vi "例6-18.vi"() -> ()   [LabVIEW 2019]
uses:
  <vilib>/Analysis/4window.llb/Hanning Window (DBL).vi
  <vilib>/Analysis/4window.llb/AllCosWindow (DBL).vi
  <vilib>/Analysis/NI_AALBase.lvlib
  <vilib>/Analysis/NI_AALPro.lvlib
panel:
  in  "停止":bool
  in  "信号2幅值":dbl=1.0
  in  "信号2频率":dbl=48.67
  in  "信号1幅值":dbl=0.001
  in  "信号1频率":dbl=90.2
  out "频谱图":dbl[][](graph)
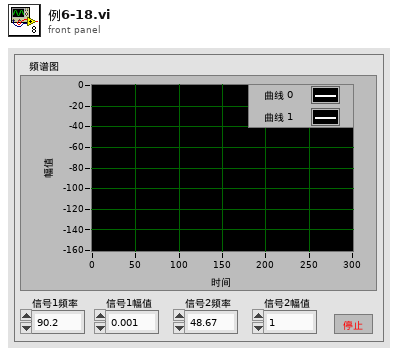
[diagram p1: front panel]
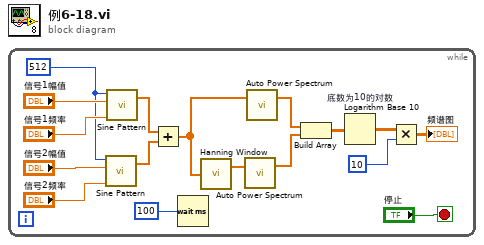
[diagram p0: block diagram]
diagram:
  n1 = while {
    stop <- "停止" stop-if-true
    w15 = 512
    n2 = call <vilib>:"Sine Pattern.vi"("cycles"="信号2频率", "amplitude"="信号2幅值", "samples"=w15) -> ("Sinusoidal Pattern"=w11:dbl[])  [unwired: 1 in, 1 out]
    n3 = call <vilib>:"Sine Pattern.vi"("cycles"="信号1频率", "amplitude"="信号1幅值", "samples"=w15) -> ("Sinusoidal Pattern"=w12:dbl[])  [unwired: 1 in, 1 out]
    n4 = Add(x=w12, y=w11) -> (x+y=w10:dbl[])
    n5 = Wait (ms)(milliseconds to wait=100) -> ()  [unwired: 1 out]
    n6 = call-poly <vilib>:"Hanning Window.vi"("X"=w10) -> ("Windowed X"=w9:dbl[])  [unwired: 1 out]
    n7 = call <vilib>:"Auto Power Spectrum.vi"("Signal (V)"=w9) -> ("Power Spectrum (V^2 rms)"=w8:dbl[])  [unwired: 1 in, 1 out]
    n8 = call <vilib>:"Auto Power Spectrum.vi"("Signal (V)"=w10) -> ("Power Spectrum (V^2 rms)"=w1:dbl[])  [unwired: 1 in, 1 out]
    n9 = Build Array(w1, w8) -> (w7:dbl[][])
    n10 = Logarithm Base 10 "底数为10的对数"(1:w7) -> (0:w6:dbl[][])
    n11 = Multiply(x=w6, y=10) -> (x*y=→"频谱图":dbl[][])
  }
